vi "TEST_DrawChecked.vi"() -> ()   [LabVIEW 2021, in "Menu.lvlib" / "Menu.lvclass"]
uses:
  Menu.lvclass
  Picture2D/src/Color/Color.lvclass
  Picture2D/src/2DPictureControl/2DPictureControl.lvclass
  Picture2D/src/PointSpecialized/PointSpecialized.lvclass
  C:/GitHub/Picture2D/src/Point/Point.lvclass
  Picture2D/src/Collection/Collection.lvclass
  C:/GitHub/Picture2D/src/IDrawable/IDrawable.lvclass
panel:
  out "2D Picture out":picture
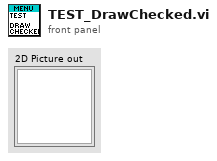
[diagram p1: front panel]
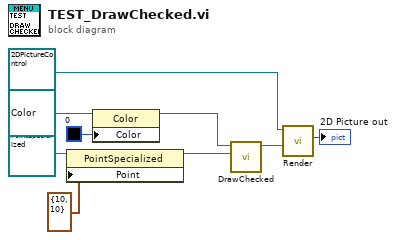
[diagram p0: block diagram]
diagram:
  n1 = property class="PointSpecialized"(reference=refnum<class "PointSpecialized.lvclass"> refnum ("Point"), "Point"=cluster{"x":i16, "y":i16} {"x"=10, "y"=10} ("Point:All Elements")) -> (reference out=w2:refnum<class "PointSpecialized.lvclass">)  [unwired: 1 in, 1 out]
  n2 = property class="Color"(reference=refnum<class "Color.lvclass"> refnum ("Color"), "Color"=u32 0) -> (reference out=w8:refnum<class "Color.lvclass">)  [unwired: 1 in, 1 out]
  n3 = call "DrawChecked.vi"("Point"=w2, "Color"=w8) -> ("Collection out"=w6:refnum<class "Collection.lvclass">)  [unwired: 8 in, 1 out]
  n4 = call-dynamic "Render.vi"("IDrawable"=w6, "2DPictureControl in"=refnum<class "2DPictureControl.lvclass"> refnum) -> ("2D Picture out"=→"2D Picture out":picture)  [unwired: 7 in, 2 out]
